vi "Save As Commented Sif.vi"(8 "error in (no error)":errorcluster, 10 "comment":string, 11 "path":string) -> (0 "error out":errorcluster, 1 "function return":u32, 2 "comment out":string, 3 "path out":string)   [LabVIEW 2014, in "atmcd32d.lvlib"]
doc: "unsigned int WINAPI SaveAsCommentedSif(char * path, char * comment);"
uses:
  atmcd32d.lvlib
  atmcd32d.dll
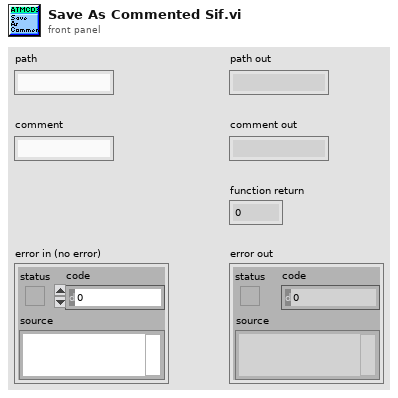
[diagram p1: front panel]
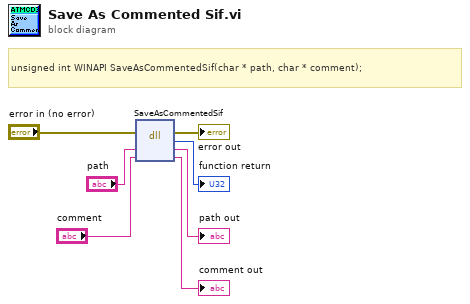
[diagram p0: block diagram]
diagram:
  # "unsigned int WINAPI SaveAsCommentedSif(char * path, char * comment);"
  n1 = dll-call lib="C:/Users/Bakir/Documents/Lambda2-Testing/lib/Andorlib/atmcd32d.*" fn="SaveAsCommentedSif"(error in="error in (no error)", "path"="path", "comment"="comment") -> (error out=→"error out":errorcluster, →"function return":u32, "path"=→"path out":string, "comment"=→"comment out":string)  [unwired: 2 in, 1 out]
